vi "think_and_act._1vi.vi"(8 "error in (no error)":errorcluster, 9 "antState":T1, 10 "pieceOfWorld":T4[][](array[typedef]), 11 "Igor in":refnum<class "Igor.lvclass">) -> (0 "error out":errorcluster, 2 "action":T2, 3 "Igor out":refnum<class "Igor.lvclass">)   [LabVIEW 2015]
doc: "Ant thinks and chooses action\nCreated by Artem Shevelev\nshevelev.pro\nartem@shevelev.pro\nLabVIEW Portal: https://labviewportal.org/memberlist.php?mode=viewprofile&u=2340"
uses:
  ant_base/ant_base.lvclass
  ant_base/actionType_enum.ctl
  ant_base/action_cluster.ctl
  actors/world/typedefs/markValue.ctl
  actors/world/world.lvlib
  actors/world/typedefs/anthillType_enum.ctl
  Igor.lvclass
  az_to_rad/az_to_rad_back.vi
  az_to_rad/az_to_rad_straight.vi
  actors/world/typedefs/amountOfFood.ctl
  actors/world/typedefs/markValue_cluster.ctl
  actors/world/typedefs/worldCell_cluster.ctl
  ant_base/antState_cluster.ctl
  actors/world/typedefs/markVolume.ctl
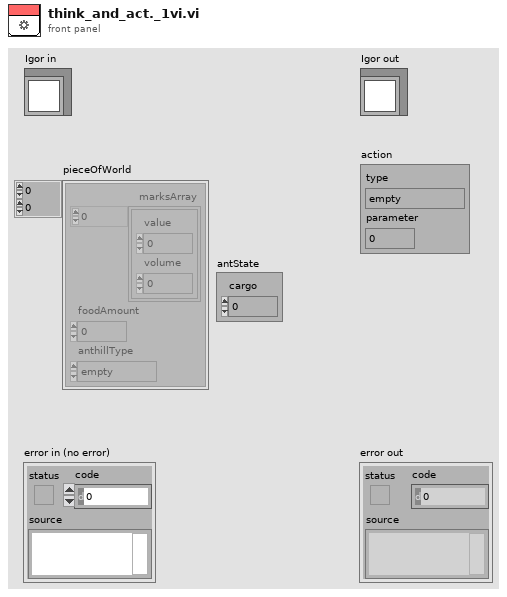
[diagram p1: front panel]
types:
  T1 = typedef "ant_base.lvclass/antState_cluster.ctl" = cluster{"cargo":u8}
  T2 = typedef "ant_base.lvclass/action_cluster.ctl" = cluster{"type":T3, "parameter":dbl}
  T3 = typedef "ant_base.lvclass/actionType_enum.ctl" = enum8{"empty", "move", "take", "put", "mark"}
  T4 = typedef "world.lvlib/worldCell_cluster.ctl" = cluster{"marksArray":T5[], "foodAmount":T8, "anthillType":T9}
  T5 = typedef "world.lvlib/markValue_cluster.ctl" = cluster{"value":T6, "volume":T7}
  T6 = typedef "world.lvlib/markValue.ctl" = u8
  T7 = typedef "world.lvlib/markVolume.ctl" = u16
  T8 = typedef "world.lvlib/amountOfFood.ctl" = i32
  T9 = typedef "world.lvlib/anthillType_enum.ctl" = enum16{"empty", "own", "rival"}
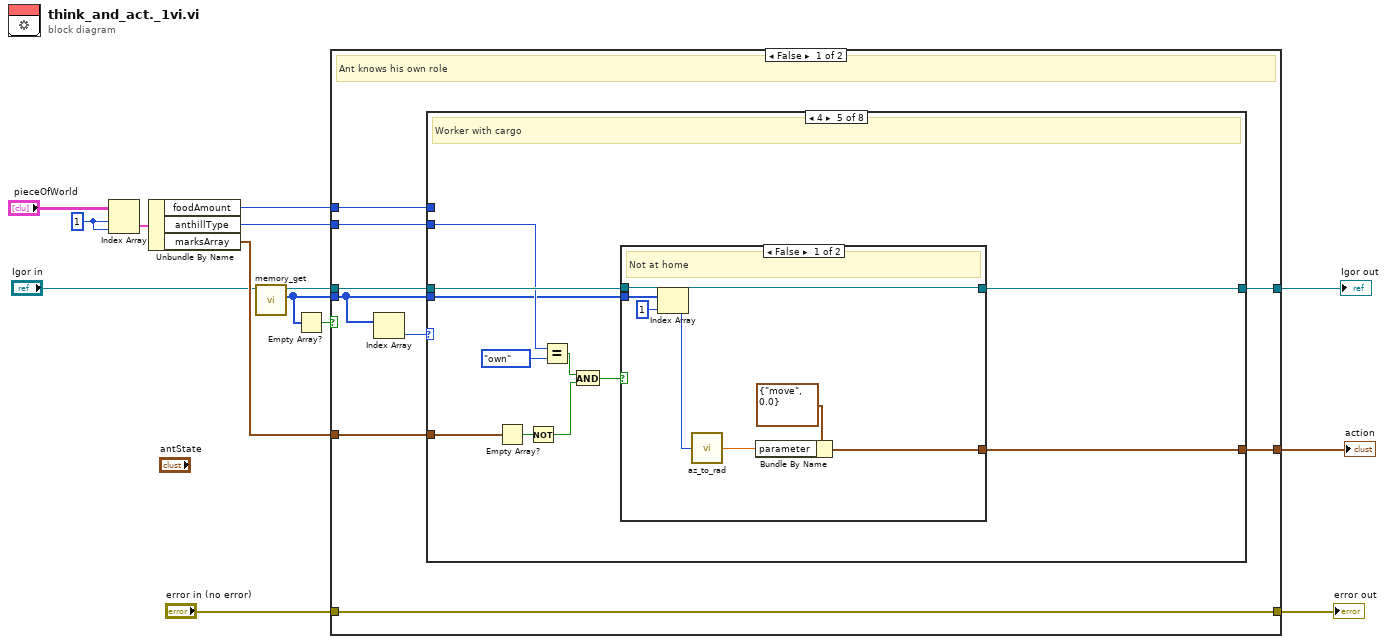
[diagram p0: block diagram]
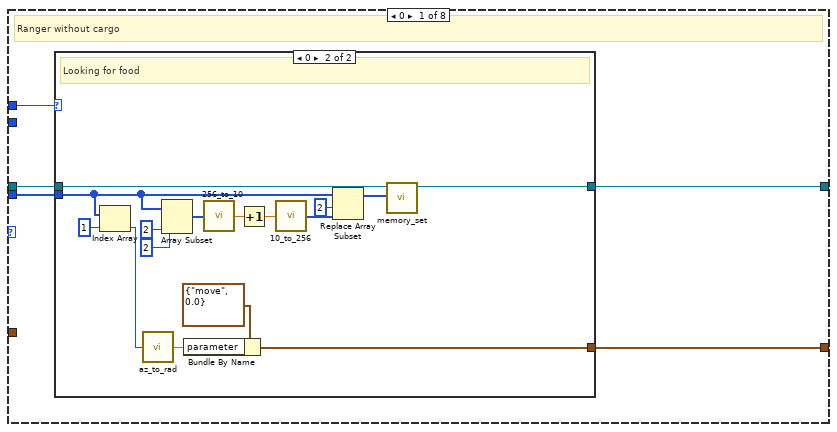
[diagram p2: hidden frame]
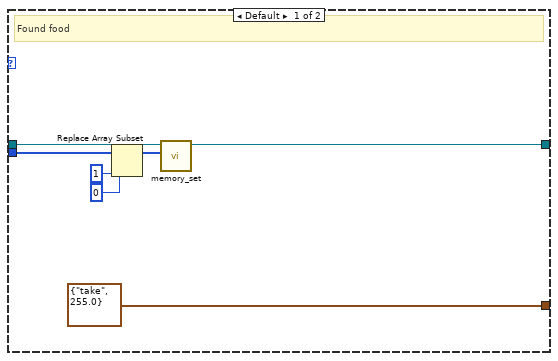
[diagram p3: hidden frame]
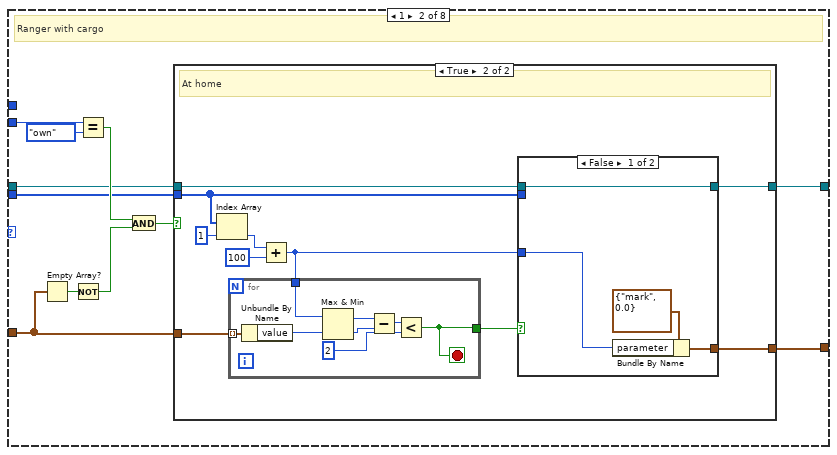
[diagram p4: hidden frame]
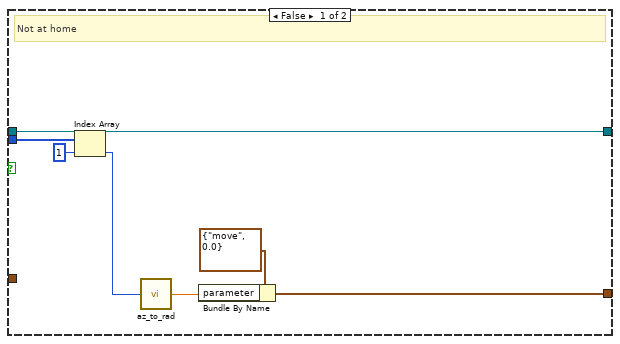
[diagram p5: hidden frame]
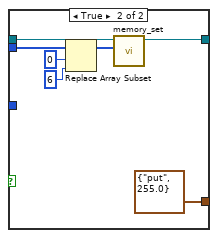
[diagram p6: hidden frame]
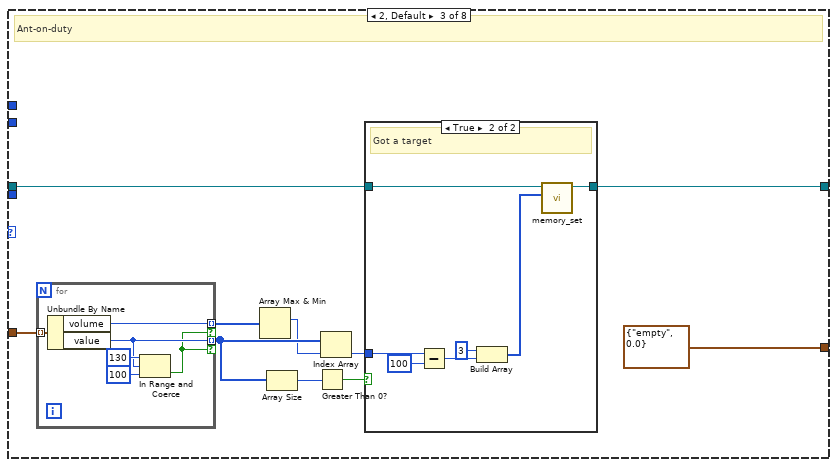
[diagram p7: hidden frame]
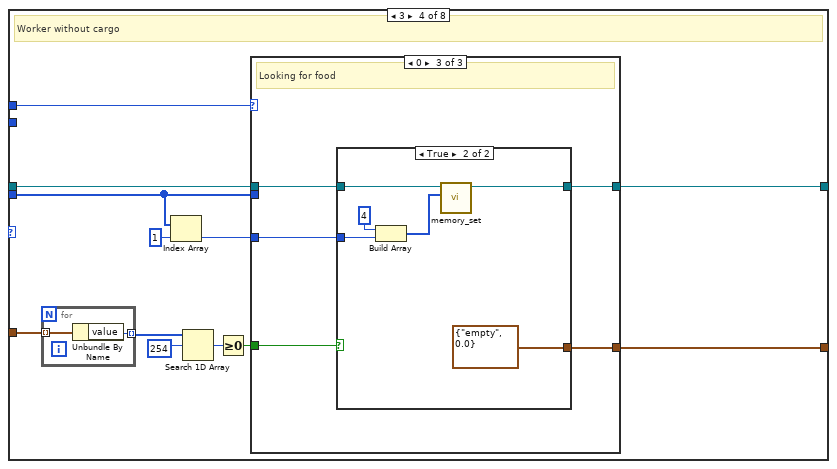
[diagram p9: hidden frame]
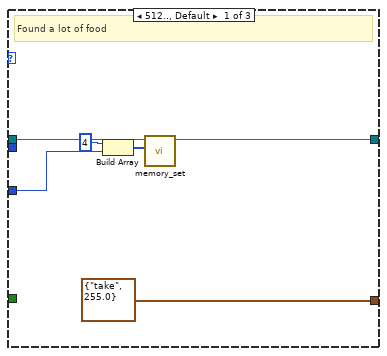
[diagram p10: hidden frame]
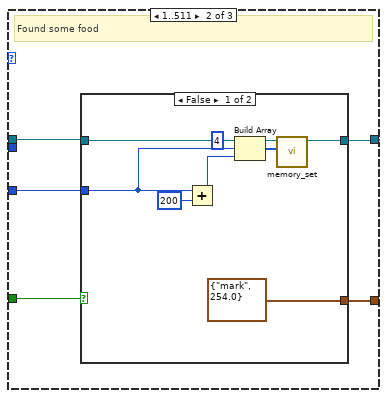
[diagram p11: hidden frame]
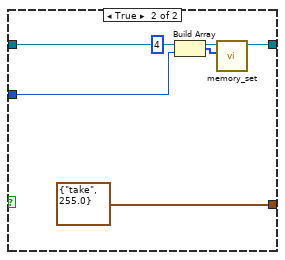
[diagram p12: hidden frame]
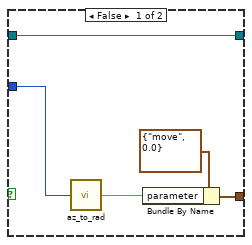
[diagram p13: hidden frame]
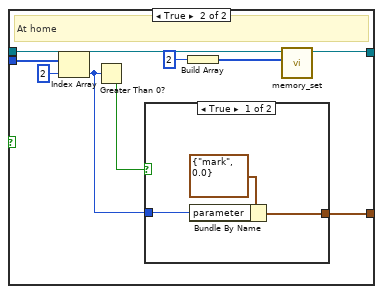
[diagram p14: hidden frame]
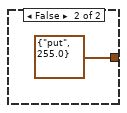
[diagram p15: hidden frame]
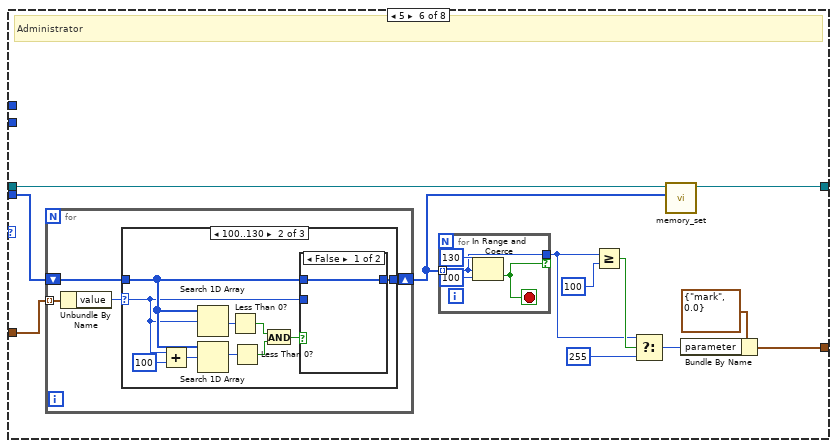
[diagram p16: hidden frame]
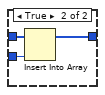
[diagram p18: hidden frame]
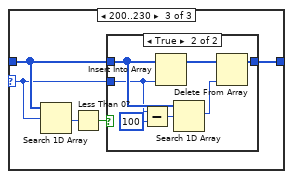
[diagram p19: hidden frame]
diagram:
  w14 = 1 ("index (row)")
  n1 = Index Array(array="pieceOfWorld", index (row)=w14, index (col)=w14) -> (element=w13:T4)
  n2 = Unbundle By Name(w13) -> ("foodAmount"=w2:T8, "anthillType"=w1:T9, "marksArray"=w7:T5[])
  n3 = call "memory_get.vi"("ant_base in"="Igor in") -> ("memory"=w3:u8[], "ant_base out"=w5:refnum<class "Igor.lvclass">)  [unwired: 8 in, 1 out]
  n4 = Empty Array?(array=w3) -> (empty?=w4:bool)
  n5 = case shown="False" w4 {
    tunnel: [w17 w364] -> w11
    tunnel: [w23 w360] -> w10
    tunnel: [w21 w358] -> w9
    tunnel: w5 -> [w18 w363]
    tunnel: "error in (no error)" -> [w23 w360]
    tunnel: w7 -> [w16 w362]
    tunnel: w3 -> [w15 _]
    tunnel: w2 -> [w20 _]
    tunnel: w1 -> [w19 _]
    frame False {
      # "Ant knows his own role"
      n6 = Index Array(array=w15) -> (element=w22:u8)  [unwired: 1 in]
      n7 = case shown="4" w22 {
        tunnel: [w28 w62 T2 {"type"=enum."empty", "parameter"=0.0} ("action") w132 w184 w220 w258 w307] -> w21
        tunnel: w20 -> [w27 _ _ w131 _ _ w259 _]
        tunnel: w19 -> [_ w61 _ _ w185 _ _ w312]
        tunnel: w18 -> [w26 w55 w106 w133 w186 w219 w261 w310]
        tunnel: [w25 w54 w107 w134 w187 w218 w270 w308] -> w17
        tunnel: w16 -> [_ w53 w108 w130 w188 w213 _ w311]
        tunnel: w15 -> [w24 w52 _ w124 w183 w212 w260 w309]
        frame 0 {
          # "Ranger without cargo"
          n8 = case shown="0" w27 {
            tunnel: [T2 {"type"=enum."take", "parameter"=255.0} ("action") w50] -> w28
            tunnel: w26 -> [w35 w40]
            tunnel: [w34 w49] -> w25
            tunnel: w24 -> [w33 w38]
            frame Default {
              # "Found food"
              n9 = Replace Array Subset(array=w33, new element=u8 1 ("new element/subarray"), index=0) -> (w32:u8[])
              n10 = call "memory_set.vi"("memory"=w32, "ant_base in"=w35) -> ("ant_base out"=w34:refnum<class "Igor.lvclass">)  [unwired: 8 in, 1 out]
            }
            frame 0 {
              # "Looking for food"
              n11 = Index Array(array=w38, index=1) -> (element=w37:u8)
              n12 = call-poly "az_to_rad.vi"("az"=w37) -> ("rad"=w39:dbl)
              n13 = Array Subset(array=w38, index=2, length=2) -> (w44:u8[])
              n14 = Bundle By Name(cluster=T2 {"type"=enum."move", "parameter"=0.0} ("action"), "parameter"=w39) -> (w50:T2)
              n15 = call "256_to_10.vi"("Array"=w44) -> ("Numeric"=w43:dbl)
              n16 = Increment(x=w43) -> (x+1=w42:dbl)
              n17 = call "10_to_256.vi"("Decimal"=w42) -> ("256"=w41:u8[])
              n18 = Replace Array Subset(array=w38, new element=w41, index=2) -> (w47:u8[])
              n19 = call "memory_set.vi"("memory"=w47, "ant_base in"=w40) -> ("ant_base out"=w49:refnum<class "Igor.lvclass">)  [unwired: 8 in, 1 out]
            }
          }
        }
        frame 1 {
          # "Ranger with cargo"
          n20 = Empty Array?(array=w53) -> (empty?=w58:bool)
          n21 = Not(x=w58) -> (.not. x?=w57:bool)
          n22 = Equal?(x=w61, y=anthillType_enum."own") -> (x = y?=w59:bool)
          n23 = And(x=w59, y=w57) -> (x .and. y?=w56:bool)
          n24 = case shown="True" w56 {
            tunnel: [w68 w75] -> w62
            tunnel: w55 -> [w67 w74]
            tunnel: [w67 w73] -> w54
            tunnel: w53 -> [_ w76]
            tunnel: w52 -> [w64 w71]
            frame False {
              # "Not at home"
              n25 = Index Array(array=w64, index=1) -> (element=w63:u8)
              n26 = call-poly "az_to_rad.vi"("az"=w63) -> ("rad"=w66:dbl)
              n27 = Bundle By Name(cluster=T2 {"type"=enum."move", "parameter"=0.0} ("action"), "parameter"=w66) -> (w68:T2)
            }
            frame True {
              # "At home"
              n28 = Index Array(array=w71, index=1) -> (element=w70:u8)
              n29 = Add(x=w70, y=u8 100) -> (x+y=w78:u8)
              n30 = for {
                tunnel: w76 -> [w98] mode=indexing
                tunnel: w78 -> [w92]
                tunnel: [w91] -> w77
                stop <- w91 stop-if-true
                n31 = Unbundle By Name(w98) -> ("value"=w93:T6)
                n32 = Max & Min(x=w92, y=w93) -> (max(x,y)=w97:T6, min(x,y)=w96:u8)
                n33 = Subtract(x=w97, y=w96) -> (x-y=w95:T6)
                n34 = Less?(x=w95, y=T6 2) -> (x < y?=w91:bool)
              }
              n35 = case shown="False" w77 {
                tunnel: [w83 T2 {"type"=enum."put", "parameter"=255.0} ("action")] -> w75
                tunnel: w78 -> [w81 _]
                tunnel: w74 -> [w80 w89]
                tunnel: [w80 w88] -> w73
                tunnel: w71 -> [_ w87]
                frame False {
                  n36 = Bundle By Name(cluster=T2 {"type"=enum."mark", "parameter"=0.0} ("action"), "parameter"=w81) -> (w83:T2)
                }
                frame True {
                  n37 = Replace Array Subset(array=w87, new element=u8 6 ("new element/subarray"), index=0) -> (w86:u8[])
                  n38 = call "memory_set.vi"("memory"=w86, "ant_base in"=w89) -> ("ant_base out"=w88:refnum<class "Igor.lvclass">)  [unwired: 8 in, 1 out]
                }
              }
            }
          }
        }
        frame 2, Default {
          # "Ant-on-duty"
          n39 = for {
            tunnel: w108 -> [w112] mode=indexing
            tunnel: [w110] -> w102 mode=indexing if=w109
            tunnel: [w111] -> w104 mode=indexing if=w109
            n40 = Unbundle By Name(w112) -> ("volume"=w111:T7, "value"=w110:T6)
            n41 = In Range and Coerce(upper limit=T6 130, x=w110, lower limit=T6 100) -> (In Range?=w109:bool)  [unwired: 1 out]
          }
          n42 = Array Max & Min(array=w104) -> (max index (indices)=w99:i32)  [unwired: 3 out]
          n43 = Array Size(array=w102) -> (size(s)=w101:i32)
          n44 = Greater Than 0?(x=w101) -> (x > 0?=w100:bool)
          n45 = Index Array(array=w102, index=w99) -> (element=w103:T6)
          n46 = case shown="True" w100 {
            tunnel: [w115 w122] -> w107
            tunnel: w106 -> [w115 w121]
            tunnel: w103 -> [_ w118]
            frame False {
              # "Expecting a target"
            }
            frame True {
              # "Got a target"
              n47 = Subtract(x=w118, y=T6 100) -> (x-y=w116:T6)
              n48 = Build Array(T6 3 ("element"), w116) -> (w120:T6[])
              n49 = call "memory_set.vi"("memory"=w120, "ant_base in"=w121) -> ("ant_base out"=w122:refnum<class "Igor.lvclass">)  [unwired: 8 in, 1 out]
            }
          }
        }
        frame 3 {
          # "Worker without cargo"
          n50 = for {
            tunnel: w130 -> [w136] mode=indexing
            tunnel: [w135] -> w129 mode=indexing
            n51 = Unbundle By Name(w136) -> ("value"=w135:T6)
          }
          n52 = Index Array(array=w124, index=1) -> (element=w123:u8)
          n53 = Search 1D Array(1D array=w129, element=T6 254) -> (index of element=w127:i32)  [unwired: 1 in]
          n54 = Greater Or Equal To 0?(x=w127) -> (x >= 0?=w126:bool)
          n55 = case shown="0" w131 {
            tunnel: w123 -> [w140 w144 w162]
            tunnel: [T2 {"type"=enum."take", "parameter"=255.0} ("action") w147 w166] -> w132
            tunnel: w133 -> [w142 w146 w164]
            tunnel: [w141 w145 w163] -> w134
            tunnel: w124 -> [_ _ _]
            tunnel: w126 -> [_ w143 w165]
            frame 512.., Default {
              # "Found a lot of food"
              n56 = Build Array(4 ("index"), w140) -> (w138:i32[])
              n57 = call "memory_set.vi"("memory"=w138, "ant_base in"=w142) -> ("ant_base out"=w141:refnum<class "Igor.lvclass">)  [unwired: 8 in, 1 out]
            }
            frame 1..511 {
              # "Found some food"
              n58 = case shown="False" w143 {
                tunnel: [T2 {"type"=enum."mark", "parameter"=254.0} ("action") T2 {"type"=enum."take", "parameter"=255.0} ("action")] -> w147
                tunnel: w146 -> [w155 w161]
                tunnel: [w154 w160] -> w145
                tunnel: w144 -> [w153 w159]
                frame False {
                  n59 = Add(x=w153, y=u8 200) -> (x+y=w150:u8)
                  n60 = Build Array(4 ("index"), w153, w150) -> (w149:i32[])
                  n61 = call "memory_set.vi"("memory"=w149, "ant_base in"=w155) -> ("ant_base out"=w154:refnum<class "Igor.lvclass">)  [unwired: 8 in, 1 out]
                }
                frame True {
                  n62 = Build Array(4 ("index"), w159) -> (w157:i32[])
                  n63 = call "memory_set.vi"("memory"=w157, "ant_base in"=w161) -> ("ant_base out"=w160:refnum<class "Igor.lvclass">)  [unwired: 8 in, 1 out]
                }
              }
            }
            frame 0 {
              # "Looking for food"
              n64 = case shown="True" w165 {
                tunnel: w162 -> [w168 w172]
                tunnel: [w170 T2 {"type"=enum."empty", "parameter"=0.0} ("action")] -> w166
                tunnel: w164 -> [w169 w177]
                tunnel: [w169 w174] -> w163
                frame False {
                  n65 = call-poly "az_to_rad.vi"("az"=w168) -> ("rad"=w167:dbl)
                  n66 = Bundle By Name(cluster=T2 {"type"=enum."move", "parameter"=0.0} ("action"), "parameter"=w167) -> (w170:T2)
                }
                frame True {
                  n67 = Build Array(T6 4 ("element"), w172) -> (w176:T6[])
                  n68 = call "memory_set.vi"("memory"=w176, "ant_base in"=w177) -> ("ant_base out"=w174:refnum<class "Igor.lvclass">)  [unwired: 8 in, 1 out]
                }
              }
            }
          }
        }
        frame 4 {
          # "Worker with cargo"
          n69 = Empty Array?(array=w188) -> (empty?=w180:bool)
          n70 = Not(x=w180) -> (.not. x?=w179:bool)
          n71 = Equal?(x=w185, y=anthillType_enum."own") -> (x = y?=w181:bool)
          n72 = And(x=w181, y=w179) -> (x .and. y?=w178:bool)
          n73 = case shown="False" w178 {
            tunnel: [w194 w197] -> w184
            tunnel: w186 -> [w193 w203]
            tunnel: [w193 w202] -> w187
            tunnel: w183 -> [w190 w201]
            frame False {
              # "Not at home"
              n74 = Index Array(array=w190, index=1) -> (element=w189:u8)
              n75 = call-poly "az_to_rad.vi"("az"=w189) -> ("rad"=w192:dbl)
              n76 = Bundle By Name(cluster=T2 {"type"=enum."move", "parameter"=0.0} ("action"), "parameter"=w192) -> (w194:T2)
            }
            frame True {
              # "At home"
              n77 = Index Array(array=w201, index=2) -> (element=w198:u8)
              n78 = Greater Than 0?(x=w198) -> (x > 0?=w199:bool)
              n79 = case shown="True" w199 {
                tunnel: w198 -> [w206 _]
                tunnel: [w205 T2 {"type"=enum."put", "parameter"=255.0} ("action")] -> w197
                frame True {
                  n80 = Bundle By Name(cluster=T2 {"type"=enum."mark", "parameter"=0.0} ("action"), "parameter"=w206) -> (w205:T2)
                }
                frame False {
                }
              }
              n81 = Build Array(u8 2 ("y")) -> (w204:u8[])
              n82 = call "memory_set.vi"("memory"=w204, "ant_base in"=w203) -> ("ant_base out"=w202:refnum<class "Igor.lvclass">)  [unwired: 8 in, 1 out]
            }
          }
        }
        frame 5 {
          # "Administrator"
          n83 = for {
            tunnel: w213 -> [w228] mode=indexing
            shift-right: [w225] -> w211
            shift-left: w212 -> [w227]
            n84 = Unbundle By Name(w228) -> ("value"=w226:T6)
            n85 = case shown="100..130" w226 {
              selector: w226 -> [_ w230 w245]
              tunnel: w227 -> [w229 w233 w247]
              tunnel: [w229 w232 w246] -> w225
              frame 0, Default {
              }
              frame 100..130 {
                n86 = Add(x=w230, y=T6 100) -> (x+y=w238:T6)
                n87 = Search 1D Array(1D array=w233, element=w230) -> (index of element=w239:i32)  [unwired: 1 in]
                n88 = Search 1D Array(1D array=w233, element=w238) -> (index of element=w235:i32)  [unwired: 1 in]
                n89 = Less Than 0?(x=w239) -> (x < 0?=w236:bool)
                n90 = Less Than 0?(x=w235) -> (x < 0?=w234:bool)
                n91 = And(x=w236, y=w234) -> (x .and. y?=w231:bool)
                n92 = case shown="False" w231 {
                  tunnel: w233 -> [w240 w243]
                  tunnel: [w240 w242] -> w232
                  tunnel: w230 -> [_ w241]
                  frame False {
                  }
                  frame True {
                    n93 = Insert Into Array(array=w243, new element=w241) -> (w242:u8[])  [unwired: 1 in]
                  }
                }
              }
              frame 200..230 {
                n94 = Search 1D Array(1D array=w247, element=w245) -> (index of element=w248:i32)  [unwired: 1 in]
                n95 = Less Than 0?(x=w248) -> (x < 0?=w244:bool)
                n96 = case shown="True" w244 {
                  tunnel: w247 -> [w249 w254]
                  tunnel: [w249 w252] -> w246
                  tunnel: w245 -> [_ w251]
                  frame False {
                  }
                  frame True {
                    n97 = Subtract(x=w251, y=T6 100) -> (x-y=w256:T6)
                    n98 = Insert Into Array(array=w254, new element=w251) -> (w253:u8[])  [unwired: 1 in]
                    n99 = Search 1D Array(1D array=w254, element=w256) -> (index of element=w250:i32)  [unwired: 1 in]
                    n100 = Delete From Array(array=w253, index=w250) -> (array with subset deleted=w252:u8[])  [unwired: 1 in, 1 out]
                  }
                }
              }
            }
          }
          n101 = for {
            tunnel: w211 -> [w222] mode=indexing
            tunnel: [w222] -> w210 if=w221
            stop <- w221 stop-if-true
            n102 = In Range and Coerce(upper limit=u8 130, x=w222, lower limit=u8 100) -> (In Range?=w221:bool)  [unwired: 1 out]
          }
          n103 = Greater Or Equal?(x=w210, y=T6 100) -> (x >= y?=w216:bool)
          n104 = Select(t=w210, s=w216, f=T6 255 ("element")) -> (s? t:f=w214:T6)
          n105 = call "memory_set.vi"("memory"=w211, "ant_base in"=w219) -> ("ant_base out"=w218:refnum<class "Igor.lvclass">)  [unwired: 8 in, 1 out]
          n106 = Bundle By Name(cluster=T2 {"type"=enum."mark", "parameter"=0.0} ("action"), "parameter"=w214) -> (w220:T2)
        }
        frame 6 {
          # "Expirienced ranger to foodHeap"
          n107 = Array Subset(array=w260, index=2, length=2 ("index")) -> (w265:u8[])
          n108 = Array Subset(array=w260, index=4, length=2) -> (w267:u8[])
          n109 = call "256_to_10.vi"("Array"=w267) -> ("Numeric"=w264:dbl)
          n110 = call "256_to_10.vi"("Array"=w265) -> ("Numeric"=w263:dbl)
          n111 = Greater Or Equal?(x=w264, y=w263) -> (x >= y?=w262:bool)
          n112 = case shown="True" w262 {
            tunnel: [w275 w303] -> w270
            tunnel: w261 -> [w276 w302]
            tunnel: w260 -> [w272 w293]
            tunnel: w259 -> [_ w291]
            tunnel: [w285 w295] -> w258
            frame False {
              # "Didn't get to foodHeap"
              n113 = Index Array(array=w272, index=1) -> (element=w271:u8)
              n114 = Array Subset(array=w272, index=4, length=2) -> (w280:u8[])
              n115 = call-poly "az_to_rad.vi"("az"=w271) -> ("rad"=w274:dbl)
              n116 = call "256_to_10.vi"("Array"=w280) -> ("Numeric"=w279:dbl)
              n117 = Bundle By Name(cluster=T2 {"type"=enum."move", "parameter"=0.0} ("action"), "parameter"=w274) -> (w285:T2)
              n118 = Increment(x=w279) -> (x+1=w278:dbl)
              n119 = call "10_to_256.vi"("Decimal"=w278) -> ("256"=w277:u8[])
              n120 = Replace Array Subset(array=w272, new element=w277, index=4) -> (w283:u8[])
              n121 = call "memory_set.vi"("memory"=w283, "ant_base in"=w276) -> ("ant_base out"=w275:refnum<class "Igor.lvclass">)  [unwired: 8 in, 1 out]
            }
            frame True {
              # "Got to foodHeap"
              n122 = Index Array(array=w293, index=1) -> (element=w292:u8)
              n123 = Greater?(x=w291, y=T8 0) -> (0:w287:bool)
              n124 = Add(x=w292, y=u8 200) -> (x+y=w289:u8)
              n125 = Select(t=u8 0 ("new element/subarray"), s=w287, f=w289) -> (s? t:f=w296:u8)
              n126 = Replace Array Subset(array=w293, new element #1=u8 7 ("new element/subarray"), index #1=0 ("index"), new element #2=w296, index #2=6 ("index")) -> (w300:u8[])
              n127 = case shown="False" w287 {
                tunnel: [T2 {"type"=enum."mark", "parameter"=254.0} ("action") T2 {"type"=enum."empty", "parameter"=0.0} ("action")] -> w295
                frame False {
                }
                frame True {
                }
              }
              n128 = call "memory_set.vi"("memory"=w300, "ant_base in"=w302) -> ("ant_base out"=w303:refnum<class "Igor.lvclass">)  [unwired: 8 in, 1 out]
            }
          }
        }
        frame 7 {
          # "Expirienced ranger from foodHeap"
          n129 = Empty Array?(array=w311) -> (empty?=w314:bool)
          n130 = Not(x=w314) -> (.not. x?=w313:bool)
          n131 = Equal?(x=w312, y=anthillType_enum."own") -> (x = y?=w315:bool)
          n132 = And(x=w315, y=w313) -> (x .and. y?=w306:bool)
          n133 = case shown="True" w306 {
            tunnel: [w322 w328] -> w307
            tunnel: w310 -> [w321 w326]
            tunnel: [w321 w327] -> w308
            tunnel: w309 -> [w318 w325]
            frame False {
              # "Not at home"
              n134 = Index Array(array=w318, index=1) -> (element=w317:u8)
              n135 = call-poly "az_to_rad.vi"("az"=w317) -> ("rad"=w320:dbl)
              n136 = Bundle By Name(cluster=T2 {"type"=enum."move", "parameter"=0.0} ("action"), "parameter"=w320) -> (w322:T2)
            }
            frame True {
              # "At home"
              n137 = Index Array(array=w325, index=6) -> (element=w324:u8)
              n138 = case shown="Default" w324 {
                selector: w324 -> [w330 _]
                tunnel: [w343 T2 {"type"=enum."empty", "parameter"=0.0} ("action")] -> w328
                tunnel: [w333 w356] -> w327
                tunnel: w326 -> [w332 w355]
                tunnel: w325 -> [w331 w354]
                frame Default {
                  n139 = Bundle By Name(cluster=T2 {"type"=enum."mark", "parameter"=0.0} ("action"), "parameter"=w330) -> (w343:T2)
                  n140 = Replace Array Subset(array=w331, new element #1=u8 0 ("new element/subarray"), index #1=0 ("index"), new element #2=u8 0 ("new element/subarray"), index #2=4 ("index"), new element #3=u8 0 ("new element/subarray"), index #3=5 ("index"), new element #4=u8 0 ("new element/subarray"), index #4=6 ("index")) -> (w334:u8[])
                  n141 = call "memory_set.vi"("memory"=w334, "ant_base in"=w332) -> ("ant_base out"=w333:refnum<class "Igor.lvclass">)  [unwired: 8 in, 1 out]
                }
                frame 0 {
                  n142 = Replace Array Subset(array=w354, new element #1=u8 6 ("new element/subarray"), index #1=0 ("index"), new element #2=u8 0 ("new element/subarray"), index #2=4 ("index"), new element #3=u8 0 ("new element/subarray"), index #3=5 ("index"), new element #4=u8 0 ("new element/subarray"), index #4=6 ("index")) -> (w345:u8[])
                  n143 = call "memory_set.vi"("memory"=w345, "ant_base in"=w355) -> ("ant_base out"=w356:refnum<class "Igor.lvclass">)  [unwired: 8 in, 1 out]
                }
              }
            }
          }
        }
      }
    }
    frame True {
      # "Ant's memory is empty"
      n144 = Delete From Array(array=w362) -> (deleted portion=w361:T5)  [unwired: 2 in, 1 out]
      n145 = Unbundle By Name(w361) -> ("value"=w359:T6)
      n146 = case shown="0..29" w359 {
        selector: w359 -> [w367 w374 w382]
        tunnel: [w372 w380 w387] -> w364
        tunnel: w363 -> [w371 w379 w386]
        tunnel: [w366 w373 w381] -> w358
        frame 0..29 {
          w365 = T6 0 ("element")
          # "Ant became a ranger"
          n147 = Increment(x=w367) -> (x+1=w368:T6)
          n148 = Build Array(w365, w367, w365, w365, w365, w365, w365) -> (w370:T6[])
          n149 = Bundle By Name(cluster=T2 {"type"=enum."mark", "parameter"=0.0} ("action"), "parameter"=w368) -> (w366:T2)
          n150 = call "memory_set.vi"("memory"=w370, "ant_base in"=w371) -> ("ant_base out"=w372:refnum<class "Igor.lvclass">)  [unwired: 8 in, 1 out]
        }
        frame 30 {
          # "Ant became an administrator"
          n151 = Increment(x=w374) -> (x+1=w375:T6)
          n152 = Build Array(T6 5 ("element")) -> (w378:T6[])
          n153 = Bundle By Name(cluster=T2 {"type"=enum."mark", "parameter"=0.0} ("action"), "parameter"=w375) -> (w373:T2)
          n154 = call "memory_set.vi"("memory"=w378, "ant_base in"=w379) -> ("ant_base out"=w380:refnum<class "Igor.lvclass">)  [unwired: 8 in, 1 out]
        }
        frame 31, Default {
          # "Ant became an ant-on-duty"
          n155 = Build Array(T6 2 ("element")) -> (w385:T6[])
          n156 = Bundle By Name(cluster=T2 {"type"=enum."mark", "parameter"=0.0} ("action"), "parameter"=w382) -> (w381:T2)
          n157 = call "memory_set.vi"("memory"=w385, "ant_base in"=w386) -> ("ant_base out"=w387:refnum<class "Igor.lvclass">)  [unwired: 8 in, 1 out]
        }
      }
    }
  }
  "error out" <- w10
  "Igor out" <- w11
  "action" <- w9
